vi "authorization_basic.vi"(8 "error in (no error)":errorcluster, 10 "password":string, 11 "username":string) -> (0 "error out":errorcluster, 3 "header":cluster{"header":string, "value":string}={"header"="Content-Type", "value"="application/json"})   [LabVIEW 2015, in "lv-dropbox.lvlib"]
uses:
  lv-dropbox.lvlib
  dependencies/dependencies.lvlib
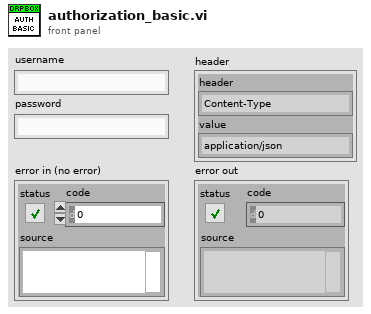
[diagram p1: front panel]
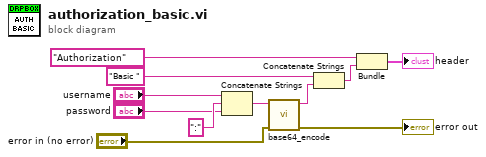
[diagram p0: block diagram]
diagram:
  n1 = Concatenate Strings("username", ":" ("string"), "password") -> (w2:string)
  n2 = call "base64_encode.vi"("error in (no error)"="error in (no error)", "string in (not encoded)"=w2) -> ("error out"=→"error out":errorcluster, "string out (base64-encoded)"=w1:string)  [unwired: 8 in]
  n3 = Concatenate Strings("Basic " ("string"), w1) -> (w8:string)
  n4 = Bundle("header"="Authorization", w8) -> (→"header":cluster{"header":string, string})  [unwired: 1 in]
